vi "SetModeConditional.vi"(0 "RobotDriveDevRef":T1={"DevStatus"={"status"=FALSE, "code"=0, "source"=""}, "Motors[]"=[], "Square Inputs"=FALSE, "Max Output"=1.0, "Isochronous"=FALSE}, 1 "P":dbl, 2 "I":dbl, 3 "D":dbl, 11 "error in (no error)":errorcluster) -> (15 "error out":errorcluster)   [LabVIEW 2013]
uses:
  <vilib>/Rock Robotics/WPI/RobotDrive/WPI_RobotDriveDevRef.ctl
  <vilib>/Rock Robotics/WPI/MotorControl/WPI_MotorControlDeviceRef.ctl
  <vilib>/Rock Robotics/SystemInterfaces/Typedef/FPGA_TypedefDigitalModule.ctl
  <vilib>/Rock Robotics/SystemInterfaces/DIO/FPGA_DIOPWMChannel.ctl
  <vilib>/Rock Robotics/WPI/PWM/WPI_PWMDeadband.ctl
  <vilib>/Rock Robotics/WPI/CAN/Jaguar/SubVIs/WPI_CANJaguar_ControlMode.ctl
  <vilib>/Rock Robotics/WPI/PWM/WPI_PWMTransform_ConPane.ctl
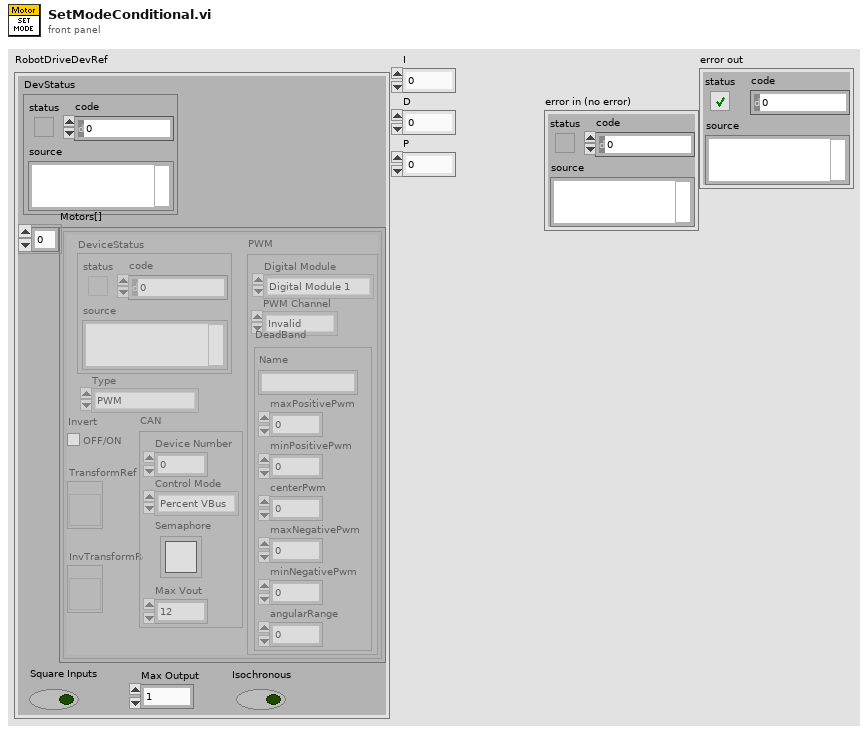
[diagram p1: front panel]
types:
  T1 = typedef "WPI_RobotDriveDevRef.ctl" = cluster{"DevStatus":errorcluster, "Motors[]":T2[], "Square Inputs":bool, "Max Output":dbl, "Isochronous":bool}
  T2 = typedef "WPI_MotorControlDeviceRef.ctl" = cluster{"DeviceStatus":errorcluster, "Type":enum16{"PWM", "CAN"}, "PWM":cluster{"Digital Module":T3, "PWM Channel":T4, "DeadBand":T5}, "CAN":cluster{"Device Number":u8, "Control Mode":T6, "Semaphore":T7, "Max Vout":dbl}, "Invert":bool, "TransformRef":T8, "InvTransformRef":T8}
  T3 = typedef "FPGA_TypedefDigitalModule.ctl" = enum16{"Digital Module 1", "Digital Module 2"}
  T4 = typedef "FPGA_DIOPWMChannel.ctl" = enum8{"PWM 1", "PWM 2", "PWM 3", "PWM 4", "PWM 5", "PWM 6", "PWM 7", "PWM 8", "PWM 9", "PWM 10", "Invalid"}
  T5 = typedef "WPI_PWMDeadband.ctl" = cluster{"Name":string, "maxPositivePwm":i32, "minPositivePwm":i32, "centerPwm":i32, "maxNegativePwm":i32, "minNegativePwm":i32, "angularRange":u16}
  T6 = typedef "WPI_CANJaguar_ControlMode.ctl" = enum8{"Percent VBus", "Current", "Speed", "Position", "Voltage"}
  T7 = typedef "Semaphore RefNum" = refnum<k1>
  T8 = typedef "WPI_PWMTransform_ConPane.ctl" = refnum<vi>
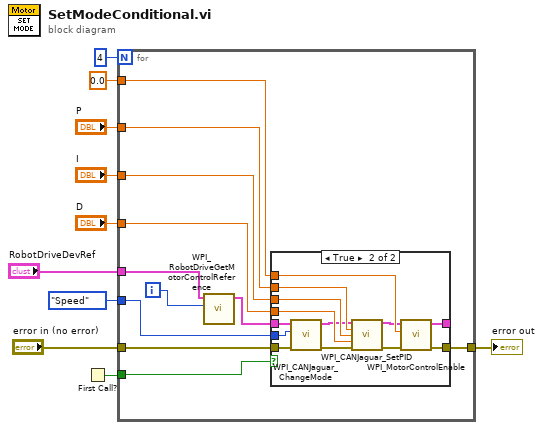
[diagram p0: block diagram]
diagram:
  n1 = First Call?() -> (First Call?: T/F=w2:bool)
  n2 = for {
    N: 4 -> [_]
    tunnel: WPI_CANJaguar_ControlMode."Speed" ("Control Mode") -> [w21]
    tunnel: 0.0 ("Encoder Initial Position") -> [w20]
    tunnel: "RobotDriveDevRef" -> [w18]
    tunnel: "error in (no error)" -> [w17]
    tunnel: "P" -> [w16]
    tunnel: "I" -> [w15]
    tunnel: "D" -> [w14]
    tunnel: [w13] -> w3
    tunnel: w2 -> [w12]
    i -> [w11]
    n3 = call <vilib>:"WPI_RobotDriveGetMotorControlReference.vi"("MotorIndex"=w11, "RobotDriveDevRef"=w18) -> ("MotorControlDeviceRef"=w19:T2)  [unwired: 9 out]
    n4 = case shown="True" w12 {
      tunnel: w20 -> [_ w36]
      tunnel: [w23 w33] -> _
      tunnel: [w22 w35] -> w13
      tunnel: w21 -> [_ w34]
      tunnel: w19 -> [w23 w29]
      tunnel: w17 -> [w22 w24]
      tunnel: w16 -> [_ w32]
      tunnel: w15 -> [_ w31]
      tunnel: w14 -> [_ w30]
      frame False {
      }
      frame True {
        n5 = call <vilib>:"WPI_CANJaguar_ChangeMode.vi"("error in (no error)"=w24, "Control Mode"=w34, "CAN Jaguar Ref"=w29) -> ("error out"=w25:errorcluster, "CAN Jaguar Ref Out"=w28:T2)  [unwired: 7 in]
        n6 = call <vilib>:"WPI_CANJaguar_SetPID.vi"("CAN Jaguar Ref"=w28, "P"=w32, "I"=w31, "D"=w30, "error in (no error)"=w25) -> ("CAN Jaguar Ref Out"=w27:T2, "error out"=w26:errorcluster)  [unwired: 9 in]
        n7 = call <vilib>:"WPI_MotorControlEnable.vi"("error in (no error)"=w26, "Encoder Initial Position"=w36, "CAN Jaguar Ref"=w27) -> ("error out"=w35:errorcluster, "CAN Jaguar Ref Out"=w33:T2)  [unwired: 7 in]
      }
    }
  }
  "error out" <- w3
